vi "编码器校准.vi"(8 "error in (no error)":errorcluster, 11 "数值":sgl) -> (0 "error out":errorcluster)   [LabVIEW 2016, in "PLC.lvlib"]
uses:
  PLC.lvlib
  <vilib>/Plasmionique/MB Master/MB_Master_Serial/MB_Master_Serial.lvclass
  C:/Program Files (x86)/National Instruments/LabVIEW 2016/vi.lib/Plasmionique/MB Master/MB_Master/MB_Master.lvclass
  <vilib>/Plasmionique/MB Master/MB Master.lvlib
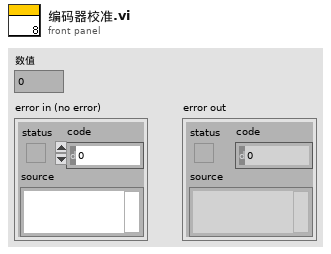
[diagram p1: front panel]
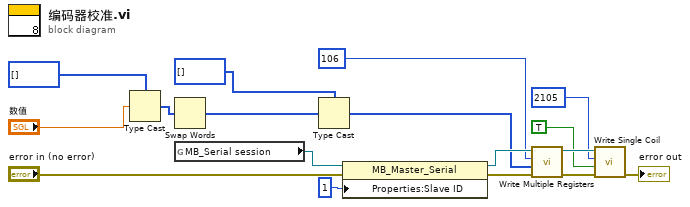
[diagram p0: block diagram]
diagram:
  n1 = Type Cast(type=u32[] [], x="数值") -> (*(type *) &x=w10:u32[])
  n2 = Swap Words(1:w10) -> (0:w9:u32[])
  n3 = global read "中间变量.vi" "MB_Serial session"() -> (w17:refnum<class "MB_Master_Serial.lvclass">)
  n4 = Type Cast(type=u16[] [], x=w9) -> (*(type *) &x=w7:u16[])
  n5 = property class="MB_Master_Serial"(reference=w17, error in="error in (no error)", "Properties:Slave ID"=u8 1 ("Slave ID")) -> (reference out=w16:refnum<class "MB_Master_Serial.lvclass">, error out=w13:errorcluster)
  n6 = call <vilib>:"Write Multiple Registers.vi"("error in (no error)"=w13, "values"=w7, "starting address"=u16 106, "MB session in"=w16) -> ("error out"=w5:errorcluster, "MB session out"=w4:refnum<class "MB_Master_Serial.lvclass">)  [unwired: 6 in]
  n7 = call <vilib>:"Write Single Coil.vi"("error in (no error)"=w5, "value"=TRUE, "address"=u16 2105, "MB session in"=w4) -> ("error out"=→"error out":errorcluster)  [unwired: 6 in, 1 out]
